vi "Set Palette Visible.vi"(6 "Control Ref Queue":T2, 8 "error in (no error)":errorcluster, 9 "Action ID in":u32=1, 10 "Item Tag":string, 11 "2D Compass.lvclass":refnum<class "2D Compass.lvclass">) -> (0 "error out":errorcluster, 1 "Action String":T1=1 items=["Show/Hide", "Change Attribute", "Text Edit", "Cursor Move"], 2 "State Change?":bool, 3 "2D Plot.lvclass out":refnum<class "2D Compass.lvclass">, 5 "Update Legend?":bool)   [LabVIEW 2017, in "2D Compass.lvclass"]
uses:
  <vilib>/Math Plots/2D Math Plots/2D Compass/2D Compass/2D Compass.lvclass
  <vilib>/Math Plots/2D Math Plots/2D Plot/Action String/2DMathPlot Ctrl Act Queue.ctl
  <vilib>/Math Plots/2D Math Plots/2D Plot/Action String/2DMathPlot Ctrl Act Cluster.ctl
  <vilib>/Math Plots/2D Math Plots/2D Plot/Action String/2DMathPlot State Class.ctl
  e:/builds/penguin/labview/branches/2017/dev/dist/vi.lib/Math Plots/2D Math Plots/2D Plot/2D Plot/2D Plot.lvclass
  <vilib>/Math Plots/2D Math Plots/2D Plot/Action String/2DMathPlot Action String.ctl
  <vilib>/Math Plots/2D Math Plots/2D Compass/2D Compass/2D Compass.lvclass/2D Compass.ctl
  <vilib>/Math Plots/2D Math Plots/2D Plot/2D Plot/2D Plot.lvclass
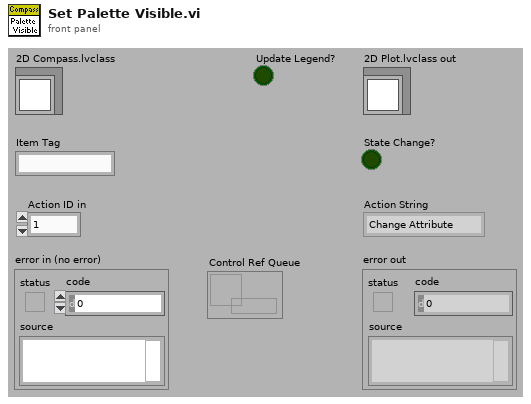
[diagram p1: front panel]
types:
  T1 = typedef "2DMathPlot Action String.ctl" = u16
  T2 = typedef "2DMathPlot Ctrl Act Queue.ctl" = refnum<queue>
  T3 = typedef "2DMathPlot Ctrl Act Cluster.ctl" = cluster{"Plot Area Ref":refnum<vi>, "Z Axis Ref":refnum<vi>, "Legend Ref":refnum<vi>, "XControl Ref":refnum<vi>, "Facade Ref":refnum<vi>, "Display State Change Class":T4}
  T4 = typedef "2DMathPlot State Class.ctl" = enum16{"Update All (Undo)", "Update General", "Update Appearance", "Update Format", "Update Scale", "Update Marker", "Update Cursor", "None"}
  T5 = typedef "2D Plot.lvclass/Property Cluster.ctl" = cluster{"Graph General":T6, "Format Property":string[], "Scale Array":T7, "Cursor Property":T10, "Annotation List":T12, "Active Cursor":i32, "Active Plot":i32}
  T6 = typedef "2D Plot.lvclass/Graph General Property.ctl" = cluster{"Palette Visible":cluster{"Graph Legend":bool, "Plot Legend":bool, "Auto size":bool, "Number of Plots":u32, "X Scrollbar":bool, "Scale Legend":bool, "Cursor Legend":bool}, "Plot Area Color":cluster{"FG Color":u32, "BG Color":u32}, "Bounds Size":cluster{"Width":u32, "Height":u32}, "Plot Area Bounds":cluster{"Left":i16, "Top":i16, "Right":i16, "Bottom":i16}}
  T7 = typedef "2D Plot.lvclass/Scale Array.ctl" = T8[]
  T8 = typedef "2D Plot.lvclass/Scale Cluster.ctl" = cluster{"General":cluster{"Editable":bool, "Flipped":bool, "Mapping Mode":u8, "Visible":bool, "Style":u8, "Scale Fit":u8}, "Offset and Multiplier":T9, "Range":cluster{"Minimum":dbl, "Maximum":dbl, "Increment":dbl, "Minor Increment":dbl, "Start":dbl}, "Tick Color":cluster{"Major Color":u32, "Minor Color":u32}, "Gird Color":cluster{"Major Color":u32, "Minor Color":u32}, "Marker":cluster{"Visible":bool, "FG Color":u32, "BG Color":u32, "Font Name":string, "Font Size":u32, "Font Bold":bool, "Font Italic":bool, "Font Strikeout":bool, "Font Underline":bool}, "Name Label":cluster{"Visible":bool, "FG Color":u32, "BG Color":u32, "Font Name":string, "Font Size":u32, "Font Bold":bool, "Font Italic":bool, "Font Strikeout":bool, "Font Underline":bool, "Justification":enum16{"Left", "Center", "Right"}, "Text":string}}
  T9 = typedef "LVOffsetAndMultiplierTypeDef.ctl" = cluster{"Offset":dbl, "Multiplier":dbl}
  T10 = typedef "2D Plot.lvclass/Cursor Property.ctl" = cluster{"Cursor List":T11, "Cursor List Addtional":cluster{"Cursor Selection Color":u32, "Line Style":u8, "Line Width":u8, "Visible":bool}[]}
  T11 = typedef "LVCursorListTypeDef.ctl" = cluster{"Name":string, "Color":u32, "Style":u8, "Point Style":u8, "Name Visible":bool, "Allow Drag":bool, "Cursor Mode":u32, "Plot":i32, "Index":i32, "Position":cluster{"X":dbl, "Y":dbl}, "X Scale":u32, "Y Scale":u32, "Watch Plots":i32[], "Watch All Plots":bool, "Plot Area":i32, "Label Offset":cluster{"X":dbl, "Y":dbl}}[]
  T12 = typedef "LVAnnotationListTypeDef.ctl" = cluster{"Name":string, "Color":u32, "Style":u8, "Point Style":u8, "Name Visible":bool, "Allow Drag":bool, "Annotation Mode":u32, "Plot":i32, "Index":i32, "Position":cluster{"X":dbl, "Y":dbl}, "X Scale":u32, "Y Scale":u32, "Show Arrow":bool, "Lock Name":bool, "Plot Area":i32, "Label Offset":cluster{"X":dbl, "Y":dbl}}[]
  T13 = typedef "LVPoint32TypeDef.ctl" = cluster{"Horizontal":i32, "Vertical":i32}
  T14 = typedef "LVRectTypeDef.ctl" = cluster{"Left":i16, "Top":i16, "Right":i16, "Bottom":i16}
  T15 = cluster{"Left":i32, "Top":i32, "Right":i32, "Bottom":i32}
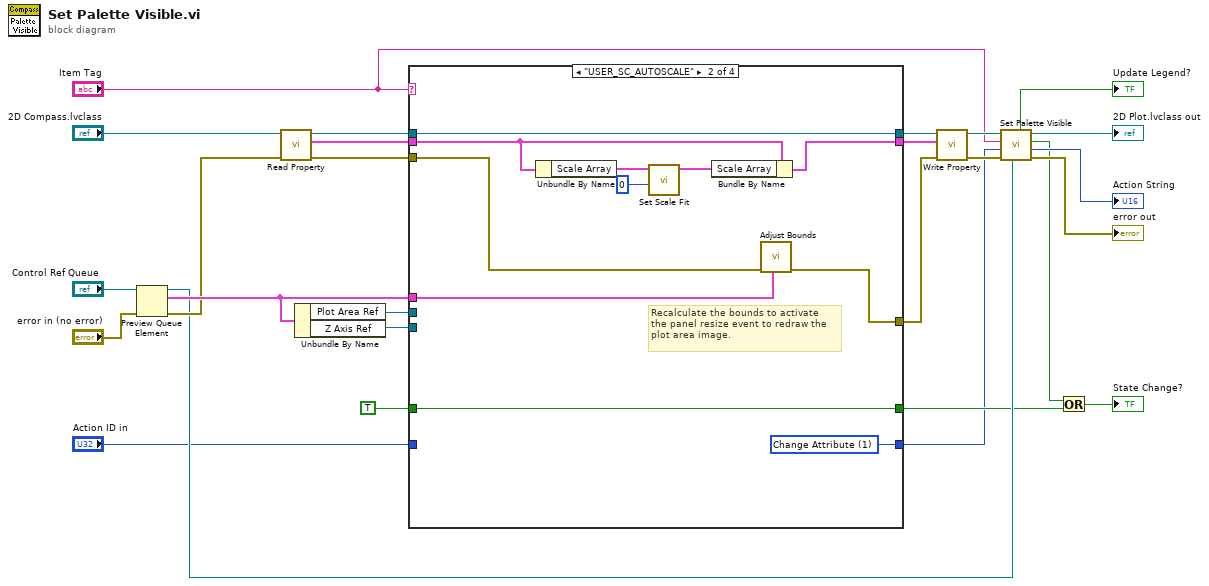
[diagram p0: block diagram]
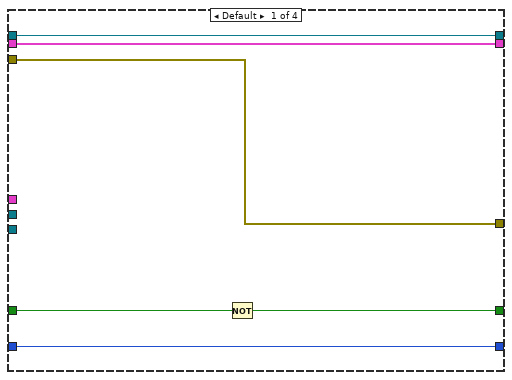
[diagram p2: hidden frame]
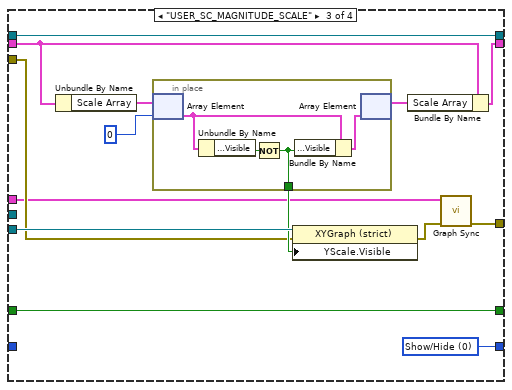
[diagram p3: hidden frame]
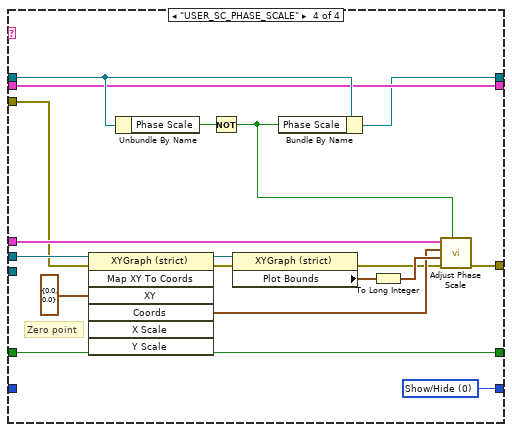
[diagram p4: hidden frame]
diagram:
  n1 = Preview Queue Element(queue="Control Ref Queue", error in (no error)="error in (no error)") -> (queue out=w10:T2, element=w18:T3, error out=w15:errorcluster)  [unwired: 2 out]
  n2 = call <vilib>:"Read Property.vi"("error in (no error)"=w15, "2D Plot.lvclass in"="2D Compass.lvclass") -> ("error out"=w23:errorcluster, "XY Graph Property Cluster"=w21:T5, "2D Plot.lvclass out"=w25:refnum<class "2D Compass.lvclass">)  [unwired: 7 out]
  n3 = Unbundle By Name(w18) -> ("Plot Area Ref"=w24:refnum<vi>, "Z Axis Ref"=w27:refnum<vi>)
  n4 = case shown="\"USER_SC_AUTOSCALE\"" "Item Tag" {
    tunnel: w21 -> [w32 w43 w56 w78]
    tunnel: [w32 w42 w55 w78] -> w20
    tunnel: w23 -> [w31 w38 w50 w65]
    tunnel: w24 -> [_ _ _ w69]
    tunnel: [w31 w37 w47 w75] -> w17
    tunnel: w25 -> [w33 w44 w57 w79]
    tunnel: [w33 w44 w57 w77] -> w26
    tunnel: w27 -> [_ _ w58 _]
    tunnel: w18 -> [_ w36 w49 w76]
    tunnel: [w29 w35 w46 w64] -> w5
    tunnel: TRUE ("State Change?") -> [w30 w35 w46 w64]
    tunnel: "Action ID in" -> [w28 _ _ _]
    tunnel: [w28 w34 w45 w63] -> w1
    frame Default {
      n5 = Not(x=w30) -> (.not. x?=w29:bool)
    }
    frame "USER_SC_AUTOSCALE" {
      w34 = T1 1 items=["Show/Hide", "Change Attribute", "Text Edit", "Cursor Move"] ("Action String in")
      # "Recalculate the bounds to activate\nthe panel resize event to redraw the \nplot area image."
      n6 = Unbundle By Name(w43) -> ("Scale Array"=w41:T7)
      n7 = call <vilib>:"Set Scale Fit.vi"("Axis Index"=0, "Scale Array In"=w41) -> ("Scale Array Out"=w40:T7)  [unwired: 9 out]
      n8 = Bundle By Name(cluster=w43, "Scale Array"=w40) -> (w42:T5)
      n9 = call <vilib>:"Adjust Bounds.vi"("Control Ref Cluster"=w36, "error in (no error)"=w38) -> ("error out"=w37:errorcluster)  [unwired: 9 out]
    }
    frame "USER_SC_MAGNITUDE_SCALE" {
      w45 = T1 0 items=["Show/Hide", "Change Attribute", "Text Edit", "Cursor Move"] ("Action String in")
      n10 = Unbundle By Name(w56) -> ("Scale Array"=w54:T7)
      n11 = in-place {
        in-place-border: [w59] -> w51
        n12 = in-place-array #1(w54, 0) -> (w61:T8)
        n13 = Unbundle By Name(w61) -> ("General.Visible"=w62:bool)
        n14 = Not(x=w62) -> (.not. x?=w59:bool)
        n15 = Bundle By Name(cluster=w61, "General.Visible"=w59) -> (w60:T8)
        n16 = in-place-array #1(w60) -> (w52:T7)  [unwired: 1 out]
      }
      n17 = property class="XYGraph (strict)"(reference=w58, error in=w50, "YScale.Visible"=w51) -> (error out=w48:errorcluster)  [unwired: 1 out]
      n18 = Bundle By Name(cluster=w56, "Scale Array"=w52) -> (w55:T5)
      n19 = call <vilib>:"Graph Sync.vi"("error in (no error)"=w48, "Control Ref Cluster"=w49) -> ("error out"=w47:errorcluster)  [unwired: 9 out]
    }
    frame "USER_SC_PHASE_SCALE" {
      w63 = T1 0 items=["Show/Hide", "Change Attribute", "Text Edit", "Cursor Move"] ("Action String in")
      # "Zero point"
      n20 = invoke on="Invoke Node" class="XYGraph (strict)" method="Map XY To Coords"(reference=w69, error in=w65, "XY"=cluster{"X":dbl, "Y":dbl} {"X"=0.0, "Y"=0.0}) -> (reference out=w73:refnum<vi>, error out=w71:errorcluster, "Coords"=w67:T13)  [unwired: 4 in, 4 out]
      n21 = Unbundle By Name(w79) -> ("Phase Scale"=w80:bool)
      n22 = Not(x=w80) -> (.not. x?=w74:bool)
      n23 = property class="XYGraph (strict)"(reference=w73, error in=w71) -> (error out=w66:errorcluster, "Plot Bounds"=w70:T14)  [unwired: 1 out]
      n24 = Bundle By Name(cluster=w79, "Phase Scale"=w74) -> (w77:refnum<class "2D Compass.lvclass">)
      n25 = To Long Integer(number=w70) -> (32bit integer=w68:T15)
      n26 = call <vilib>:"Adjust Phase Scale.vi"("Show Scale?"=w74, "error in (no error)"=w66, "Plot Area Bounds"=w68, "Origin Coords"=w67, "Control Ref Cluster"=w76) -> ("error out"=w75:errorcluster)  [unwired: 6 out]
    }
  }
  n27 = call <vilib>:"Write Property.vi"("error in (no error)"=w17, "XY Graph Property Cluster"=w20, "2D Plot.lvclass in"=w26) -> ("error out"=w12:errorcluster, "2D Plot.lvclass out"=w14:refnum<class "2D Compass.lvclass">)  [unwired: 7 out]
  n28 = call-parent "Set Palette Visible.vi"("Control Ref Queue"=w10, "error in (no error)"=w12, "Action ID in"=w1, "Item Tag"="Item Tag", "2D Plot in"=w14) -> ("error out"=→"error out":errorcluster, "Action String"=→"Action String":T1, "State Change?"=w4:bool, "2D Plot out"=→"2D Plot.lvclass out":refnum<class "2D Compass.lvclass">, "Update Legend?"=→"Update Legend?":bool)  [unwired: 2 out]
  n29 = Or(x=w4, y=w5) -> (x .or. y?=→"State Change?":bool)
